vi "Read_Code_Offset.vi"(0 "State":enum16{"Fetch", "Config+Fetch"}(ring), 1 "SYS_IMULT":u16=12, 2 "Repeat":i32=1 min=1 max=100, 5 "Port_No":u16=1444, 7 "Core_No":u16=1, 9 "ADC_Controls":T4={"ACQPS"=9, "Break_PT"=0, "Ref_Mod_Sel"=enum."Int_Ref_2P5", "Ref_Sel(Int/Ext)"=enum."Ext", "ADC"=enum."A", "Channel"=6, "LV_samples"=16384, "AGPIO_SEL"=0.0, "LV_perscale"=2}, 11 "error in":errorcluster, 12 "Refrence":dbl=2.5 format="%#_13g") -> (6 "AvgCode":dbl, 15 "error out":errorcluster)   [LabVIEW 2019]
uses:
  Ctrls/Ref_Mode_Sel.ctl
  Ctrls/Ref_Sel(Int&Ext).ctl
  Ctrls/ADC_CTRL.ctl
  <userlib>/_TI-LA/Reusable/CCS/APIs/CCS.lvlib
panel:
  out "Tot-Error":u32=4021
  out "min value":u32=33
  out "max value":u32=4054
  out "Voltage":dbl
  out "ADC_No":u16
  out "Waveform Graph":u32[](graph)
  out "Read Data[]":u32[](array[numeric]) format="%#.0f"
  # "1P65-0/2P5-1_Mode_Sel"
  # "LV_Break  = 0;\nUint16 LV_Repeat = 0;\nUint16 LV_Config = 0;\nUint16 LV_samples = 8192;\nUint16 LV_prescale = 2;\nUint16 LV_acqps = 25;\nUint16 LV_AGPIO_TEST = 0;\nUint32 LV_Avg = 0;\nUint16 LV_adcref=   1; // Internal Reference = 0\nUint16 LV_int2p5en= 1; // 2.5V Reference select = 1\nUint16 LV_adcmod =  2; // Adc sel A-0,B-1 & C-2\nUint16 LV_adcchan = 0; // Selecting ADC Channel\nUint16 LV_SYS_MULT =10;"
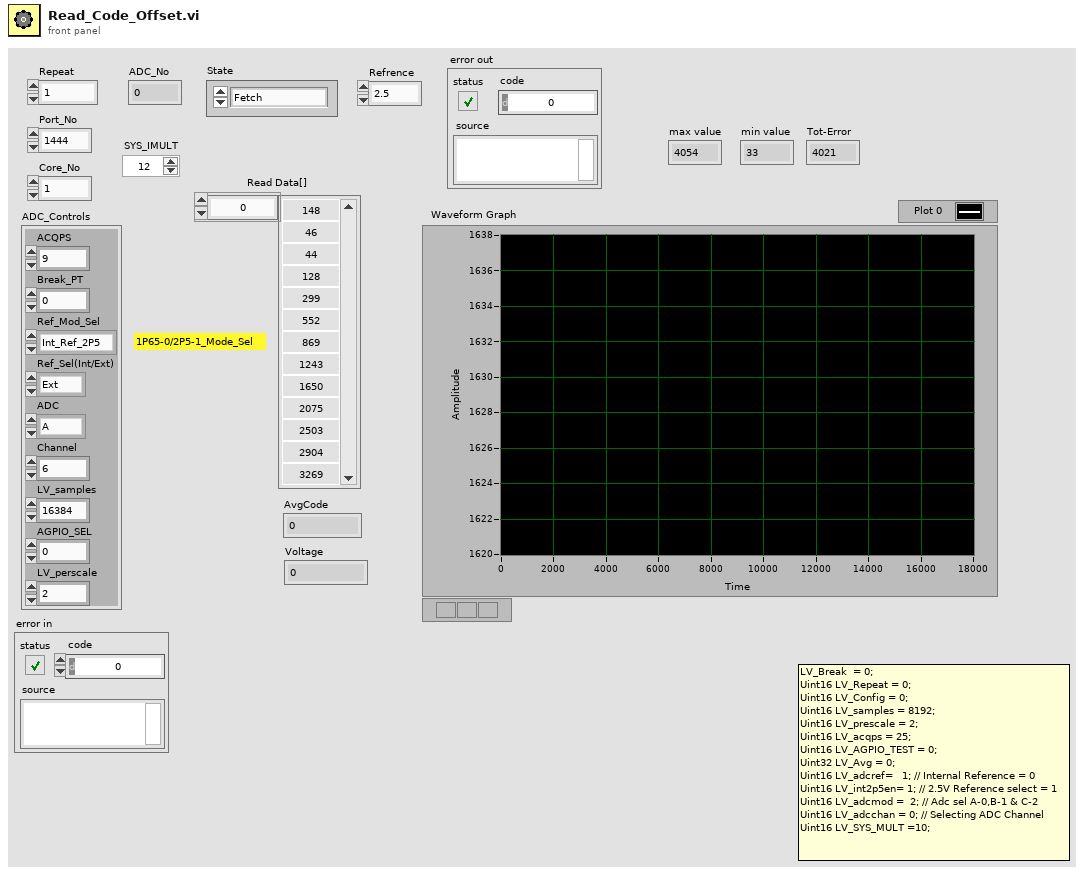
[diagram p1: front panel]
types:
  T1 = typedef "Ref_Mode_Sel.ctl" = enum16{"Int_Ref_1P65", "Int_Ref_2P5"}
  T2 = typedef "Ref_Sel(Int&Ext).ctl" = enum16{"Int", "Ext"}
  T3 = typedef "ADC_CTRL.ctl" = enum16{"A", "B", "C"}
  T4 = cluster{"ACQPS":u16, "Break_PT":u16, "Ref_Mod_Sel":T1, "Ref_Sel(Int/Ext)":T2, "ADC":T3, "Channel":u16, "LV_samples":u16, "AGPIO_SEL":dbl, "LV_perscale":u16}
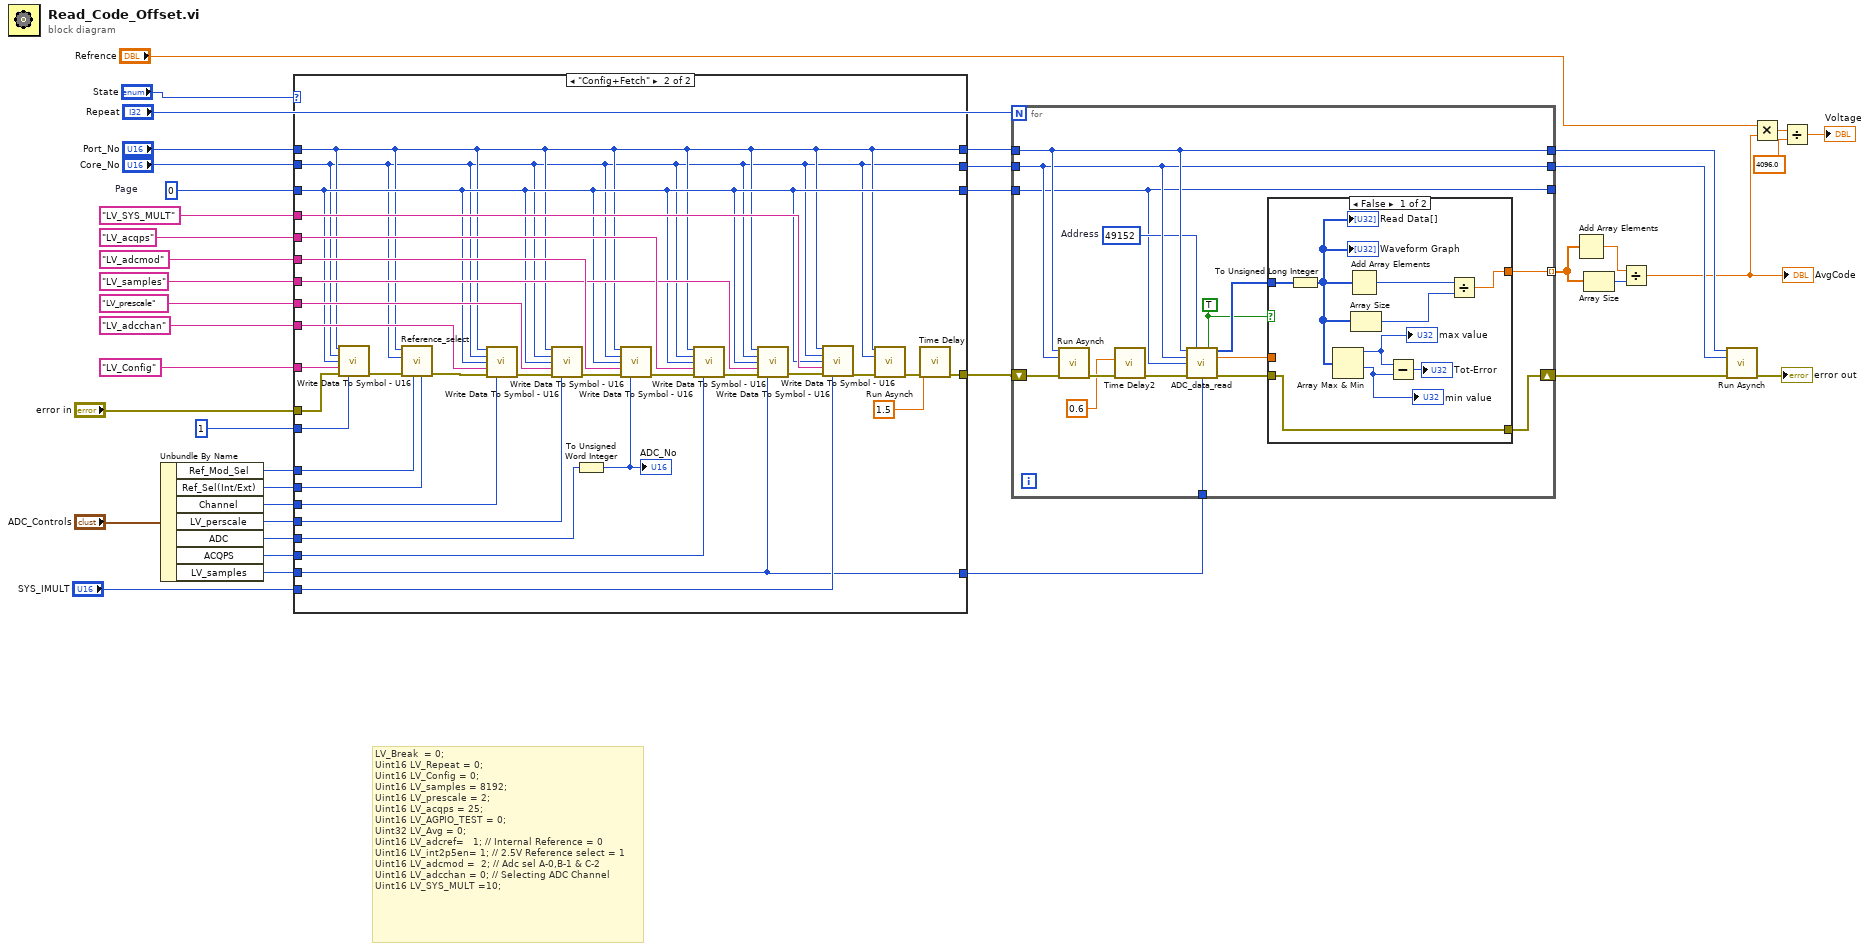
[diagram p0: block diagram]
diagram:
  w12 = 0  # Page
  # "LV_Break  = 0;\nUint16 LV_Repeat = 0;\nUint16 LV_Config = 0;\nUint16 LV_samples = 8192;\nUint16 LV_prescale = 2;\nUint16 LV_acqps = 25;\nUint16 LV_AGPIO_TEST = 0;\nUint32 LV_Avg = 0;\nUint16 LV_adcref=   1; // Internal Reference = 0\nUint16 LV_int2p5en= 1; // 2.5V Reference select = 1\nUint16 LV_adcmod =  2; // Adc sel A-0,B-1 & C-2\nUint16 LV_adcchan = 0; // Selecting ADC Channel\nUint16 LV_SYS_MULT =10;"
  n1 = Unbundle By Name("ADC_Controls") -> ("Ref_Mod_Sel"=w22:T1, "Ref_Sel(Int/Ext)"=w21:T2, "Channel"=w20:u16, "LV_perscale"=w19:u16, "ADC"=w18:T3, "ACQPS"=w17:u16, "LV_samples"=w8:u16)
  n2 = case shown="\"Config+Fetch\"" "State" {
    tunnel: "error in" -> [w45 w72]
    tunnel: "LV_Config" ("Device_No") -> [_ w71]
    tunnel: "LV_prescale" -> [_ w68]
    tunnel: "LV_adcchan" -> [_ w67]
    tunnel: "LV_adcmod" -> [_ w66]
    tunnel: "LV_acqps" -> [_ w65]
    tunnel: "LV_samples" -> [_ w64]
    tunnel: u16 1 ("Write Data") -> [_ w63]
    tunnel: w22 -> [_ w62]
    tunnel: w21 -> [_ w61]
    tunnel: w20 -> [_ w60]
    tunnel: w19 -> [_ w59]
    tunnel: w18 -> [_ w58]
    tunnel: w17 -> [_ w57]
    tunnel: [w45 w55] -> w16
    tunnel: w8 -> [w44 w49]
    tunnel: "Port_No" -> [w42 w47]
    tunnel: "Core_No" -> [w41 w46]
    tunnel: w12 -> [w43 w48]
    tunnel: "LV_SYS_MULT" -> [_ w51]
    tunnel: "SYS_IMULT" -> [_ w50]
    tunnel: [w44 w49] -> w7
    tunnel: [w43 w48] -> w3
    tunnel: [w42 w47] -> w2
    tunnel: [w41 w46] -> w1
    frame "Fetch", Default {
    }
    frame "Config+Fetch" {
      n3 = call <userlib>:"Write Data To Symbol - U16.vi"("Port Number"=w47, "Core Number"=w46, "Page"=w48, "Symbol Name"=w71, "error in"=w72, "Write Data"=w63) -> ("error out"=w70:errorcluster)  [unwired: 7 in, 2 out]
      n4 = call "Reference_select.vi"("Ref_Sel(Int/Ext)"=w61, "INT_Ref_Sel"=w62, "error in"=w70, "Core Number"=w46, "Port Number"=w47) -> ("error out"=w69:errorcluster)  [unwired: 6 in]
      n5 = call <userlib>:"Write Data To Symbol - U16.vi"("Port Number"=w47, "Core Number"=w46, "Page"=w48, "Symbol Name"=w67, "error in"=w69, "Write Data"=w60) -> ("error out"=w76:errorcluster)  [unwired: 7 in, 2 out]
      n6 = call <userlib>:"Write Data To Symbol - U16.vi"("Port Number"=w47, "Core Number"=w46, "Page"=w48, "Symbol Name"=w68, "error in"=w76, "Write Data"=w59) -> ("error out"=w75:errorcluster)  [unwired: 7 in, 2 out]
      n7 = To Unsigned Word Integer(number=w58) -> (unsigned 16bit integer=w73:u16)
      "ADC_No" <- w73
      n8 = call <userlib>:"Write Data To Symbol - U16.vi"("Port Number"=w47, "Core Number"=w46, "Page"=w48, "Symbol Name"=w66, "error in"=w75, "Write Data"=w73) -> ("error out"=w77:errorcluster)  [unwired: 7 in, 2 out]
      n9 = call <userlib>:"Write Data To Symbol - U16.vi"("Port Number"=w47, "Core Number"=w46, "Page"=w48, "Symbol Name"=w65, "error in"=w77, "Write Data"=w57) -> ("error out"=w74:errorcluster)  [unwired: 7 in, 2 out]
      n10 = call <userlib>:"Write Data To Symbol - U16.vi"("Port Number"=w47, "Core Number"=w46, "Page"=w48, "Symbol Name"=w64, "error in"=w74, "Write Data"=w49) -> ("error out"=w53:errorcluster)  [unwired: 7 in, 2 out]
      n11 = call <userlib>:"Write Data To Symbol - U16.vi"("Port Number"=w47, "Core Number"=w46, "Page"=w48, "Symbol Name"=w51, "error in"=w53, "Write Data"=w50) -> ("error out"=w52:errorcluster)  [unwired: 7 in, 2 out]
      n12 = call <userlib>:"Run Asynch.vi"("Port Number"=w47, "Core Number"=w46, "error in"=w52) -> ("error out"=w56:errorcluster)  [unwired: 10 in, 2 out]
      n13 = call "Time Delay"("error in (no error)"=w56, "Delay Time (s)"=1.5) -> ("error out"=w55:errorcluster)  [unwired: 9 in]
    }
  }
  n14 = for {
    N: "Repeat" -> [_]
    tunnel: [w92] -> w39 mode=indexing
    tunnel: w2 -> [w90]
    tunnel: w1 -> [w89]
    shift-right: [w82] -> w4
    shift-left: w16 -> [w91]
    tunnel: [w90] -> w38
    tunnel: [w89] -> w37
    tunnel: [w78] -> _
    tunnel: w7 -> [w87]
    tunnel: w3 -> [w78]
    w85 = TRUE ("Read_AVG ?")
    w86 = u32 49152  # Address
    n15 = call <userlib>:"Run Asynch.vi"("Port Number"=w90, "Core Number"=w89, "error in"=w91) -> ("error out"=w81:errorcluster)  [unwired: 10 in, 2 out]
    n16 = call "Time Delay2"("error in (no error)"=w81, "Delay Time (s)"=0.6) -> ("error out"=w80:errorcluster)  [unwired: 9 in]
    n17 = call "ADC_data_read.vi"("Port Number"=w90, "Address"=w86, "Read_AVG ?"=w85, "Core Number"=w89, "Page"=w78, "error in (no error)"=w80, "Lv_Samples"=w87) -> ("Read Data[]"=w88:u16[], "Read Data"=w84:dbl, "error out"=w83:errorcluster)  [unwired: 6 in]
    n18 = case shown="False" w85 {
      tunnel: [w100 w103] -> w92
      tunnel: w88 -> [w95 _]
      tunnel: w84 -> [_ w103]
      tunnel: w83 -> [w93 w102]
      tunnel: [w93 w102] -> w82
      frame False {
        n19 = To Unsigned Long Integer(number=w95) -> (unsigned 32bit integer=w94:u32[])
        "Waveform Graph" <- w94
        "Read Data[]" <- w94
        n20 = Array Max & Min(array=w94) -> (max value=w98:u32, min value=w97:u32)  [unwired: 2 out]
        "max value" <- w98
        "min value" <- w97
        n21 = Add Array Elements(numeric array=w94) -> (sum=w101:u32)
        n22 = Array Size(array=w94) -> (size(s)=w99:i32)
        n23 = Subtract(x=w98, y=w97) -> (x-y=→"Tot-Error":u32)
        n24 = Divide(x=w101, y=w99) -> (x/y=w100:dbl)
      }
      frame True {
      }
    }
  }
  n25 = Add Array Elements(numeric array=w39) -> (sum=w5:dbl)
  n26 = Array Size(array=w39) -> (size(s)=w6:i32)
  n27 = Divide(x=w5, y=w6) -> (x/y=w35:dbl)
  "AvgCode" <- w35
  n28 = call <userlib>:"Run Asynch.vi"("Port Number"=w38, "Core Number"=w37, "error in"=w4) -> ("error out"=→"error out":errorcluster)  [unwired: 10 in, 2 out]
  n29 = Multiply(x="Refrence", y=w35) -> (x*y=w33:dbl)
  n30 = Divide(x=w33, y=4096.0) -> (x/y=→"Voltage":dbl)
